vi "Test_StandardLogic_WriteOne_TerminalVisible.vi"(8 "error in (no error)":errorcluster, 11 "TestCase in":refnum<class "TestTerminalVisibilityBinding.lvclass">) -> (0 "error out":errorcluster, 3 "TestCase out":refnum<class "TestTerminalVisibilityBinding.lvclass">)   [LabVIEW 2017, in "TestTerminalVisibilityBinding.lvclass"]
uses:
  TestTerminalVisibilityBinding.lvclass
  Source/Concrete/TerminalVisibilityBinding/TerminalVisibilityBinding.lvclass
  C:/Git/composed-transport/Source/ITransport/ITransport.lvclass
  Source/ITransport/ITransport.lvclass
panel:
  in  "Numeric":i32
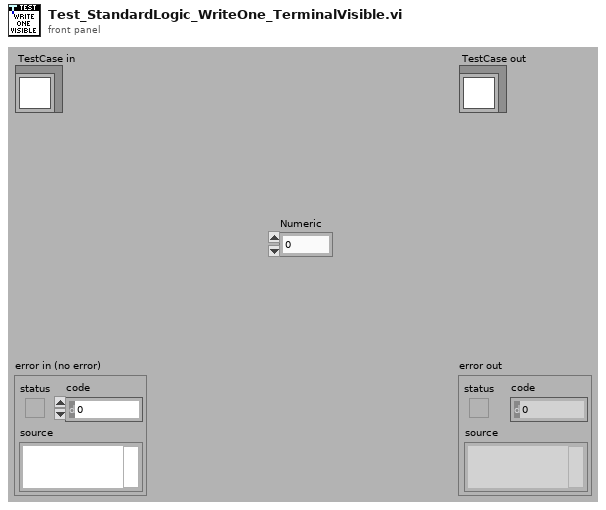
[diagram p1: front panel]
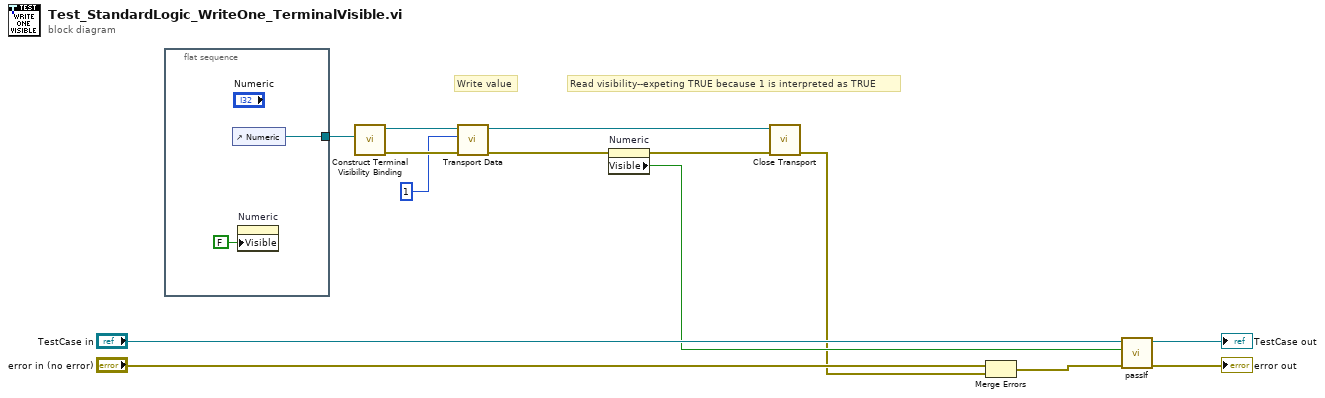
[diagram p0: block diagram]
diagram:
  # "Read visibility--expeting TRUE because 1 is interpreted as TRUE"
  # "Write value"
  n1 = flat-sequence {
    tunnel: [w16] -> w5
    frame #0 {
      n2 = control-ref of="Numeric"() -> (w16:refnum<vi>)
      n3 = property on="Numeric" class="DigNum (strict)"("Visible"=FALSE) -> ()  [unwired: 2 in, 2 out]
    }
  }
  n4 = call "Construct Terminal Visibility Binding.vi"("Ctl Refnum"=w5) -> ("error out"=w8:errorcluster, "TerminalVisibilityBinding"=w10:refnum<class "TerminalVisibilityBinding.lvclass">)  [unwired: 9 in]
  n5 = call "Transport Data.vi"("error in (no error)"=w8, "Value"=1, "ITransport in"=w10) -> ("error out"=w4:errorcluster, "ITransport out"=w6:refnum<class "TerminalVisibilityBinding.lvclass">)  [unwired: 7 in]
  n6 = property on="Numeric" class="DigNum (strict)"(error in=w4) -> (error out=w3:errorcluster, "Visible"=w2:bool)  [unwired: 1 in, 1 out]
  n7 = call-dynamic "Close Transport.vi"("error in (no error)"=w3, "ITransport in"=w6) -> ("error out"=w1:errorcluster)  [unwired: 9 in]
  n8 = Merge Errors("error in (no error)", w1) -> (w9:errorcluster)
  n9 = call-dynamic "passIf.vi"("error in (no error)"=w9, "pass"=w2, "TestCase in"="TestCase in") -> ("error out"=→"error out":errorcluster, "TestCase out"=→"TestCase out":refnum<class "TestTerminalVisibilityBinding.lvclass">)  [unwired: 7 in]
